vi "CheckVariantForClusterUpdate_HWLoop.vi"(8 "ErrorIn":errorcluster, 9 "VariantIn":variant, 11 "ClusterIn":T1={"FPGA"={"Target"=enum."4", "Channel"=enum."4", "Ref1"=refnum, "Ref2"=refnum}}) -> (0 "ErrorOut":errorcluster, 3 "ClusterOut":T1={"FPGA"={"Target"=enum."4", "Channel"=enum."4", "Ref1"=refnum, "Ref2"=refnum}})   [LabVIEW 2018]
doc: "Check the input <B>VariantIn</B> to see if it has a non-null value. If it has a valid input, convert it to a cluster and save it to <B>ClusterOut</B>, otherwise, pass <B>ClusterIn</B> straight through to <B>ClusterOut</B>.\n\nThis mechanism is useful to pass an updated cluster from one loop to another. The sending loop places a cluster as a variant into a shared queue. A receiving loop removes the element from the shared queue and checks the variant using this VI. If the variant has value, this VI replaces the receiving loop's stored cluster (usually stored via a shift register) with the cluster obtained from the variant. \n\nCopyright © 2019 Epimedia, Inc. All Rights Reserved.\n\nThe Epimedia Application Library is Copyright © 2009-2019 Epimedia, Inc. \nAll Rights Reserved. Used under license."
uses:
  Controls/HWCluster.ctl
  Controls/Clusts/FPGA_Config_Clust.ctl
  Controls/Enums/TargetNumber.ctl
panel:
  # "Copyright © 2019 Epimedia, Inc. All Rights Reserved.\n\nThe Epimedia Application Library is Copyright © 2009-2019 Epimedia, Inc. \nAll Rights Reserved. Used under license."
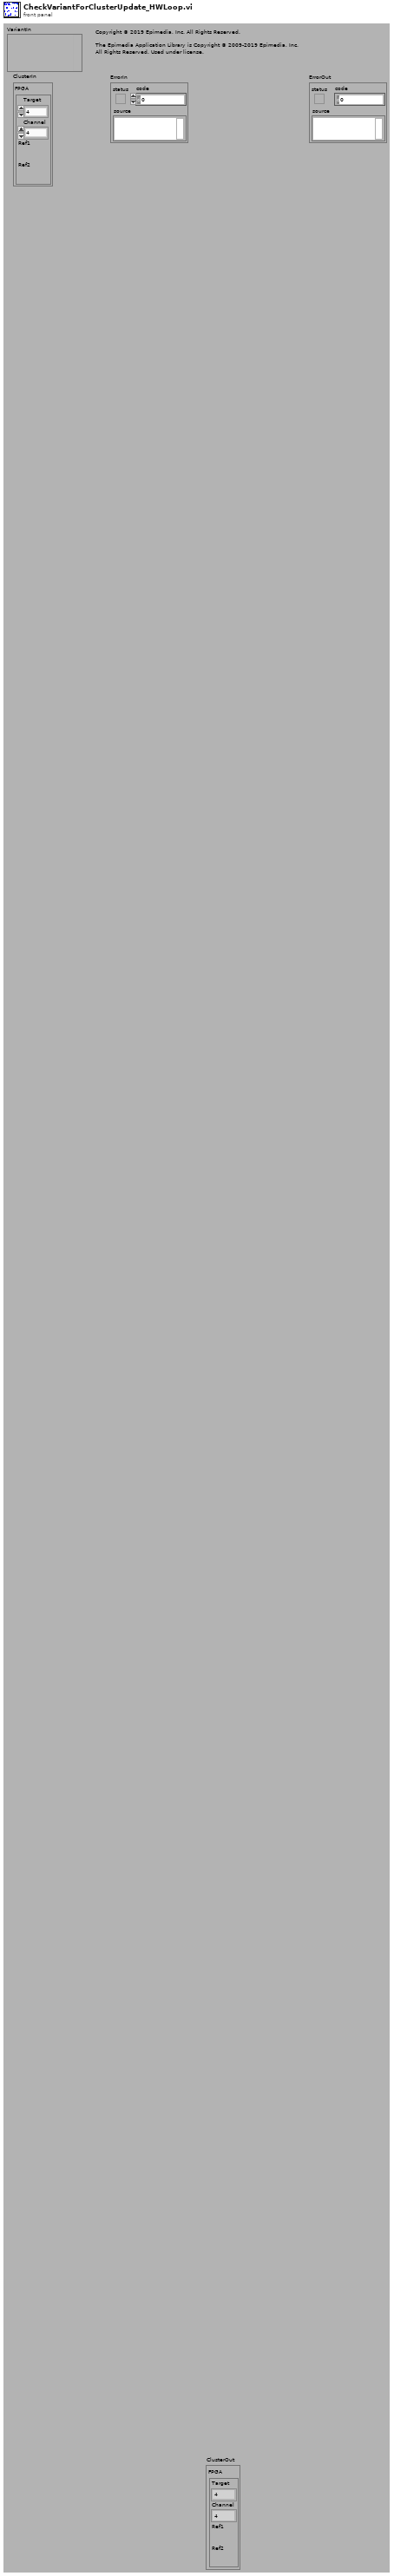
[diagram p1: front panel]
types:
  T1 = typedef "HWCluster.ctl" = cluster{"FPGA":T2}
  T2 = typedef "FPGA_Config_Clust.ctl" = cluster{"Target":T3, "Channel":T3, "Ref1":refnum<k20>, "Ref2":refnum<k20>}
  T3 = typedef "TargetNumber.ctl" = enum16{"1", "2", "3", "4"}
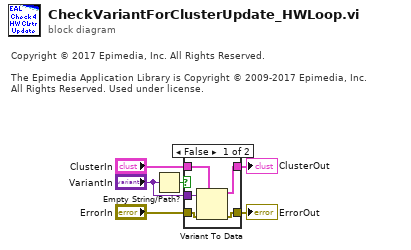
[diagram p0: block diagram]
diagram:
  # "Copyright © 2017 Epimedia, Inc. All Rights Reserved.\n\nThe Epimedia Application Library is Copyright © 2009-2017 Epimedia, Inc. \nAll Rights Reserved. Used under license."
  n1 = Empty String/Path?(string/path="VariantIn") -> (empty?=w2:bool)
  n2 = case shown="False" w2 {
    tunnel: "ErrorIn" -> [w11 w13]
    tunnel: [w10 w13] -> w6
    tunnel: "VariantIn" -> [w9 _]
    tunnel: "ClusterIn" -> [w8 w12]
    tunnel: [w7 w12] -> w5
    frame False {
      n3 = Variant To Data(error in=w11, type=w8, Variant=w9) -> (data=w7:T1, error out=w10:errorcluster)
    }
    frame True {
    }
  }
  "ErrorOut" <- w6
  "ClusterOut" <- w5
